vi "joystick+conversions.vi"(0 "Refnum in":refnum<k1>, 7 "error in (no error)":errorcluster, 8 "Stop":bool) -> (10 "dir info":i32, 12 "x axis info":i32, 13 "B pressed":bool, 14 "v_radial":dbl, 15 "y axis info":i32, 16 "A pressed":bool, 17 "y axis rot info":i32, 18 "chute":dbl, 19 "v_normal":dbl, 20 "Refnum out":refnum<k1>, 21 "X pressed":bool, 22 "R*w":dbl, 23 "Boolean":bool, 24 "z axis info (chute)":i32, 25 "Y pressed":bool, 26 "x axis rot info":i32, 27 "error out":errorcluster)   [LabVIEW 2016]
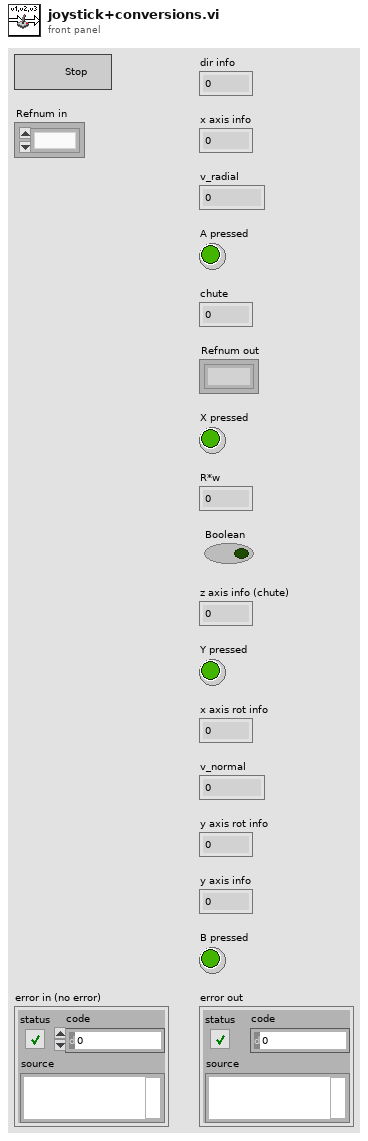
[diagram p1: front panel]
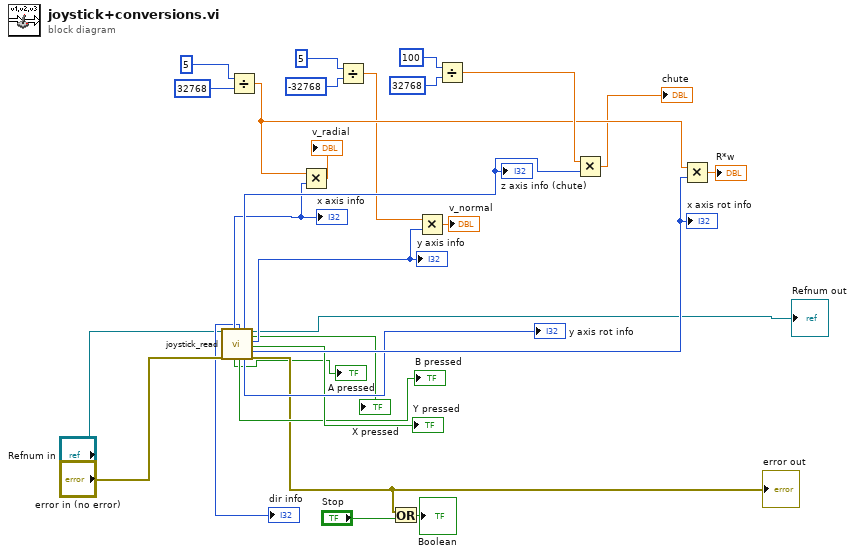
[diagram p0: block diagram]
diagram:
  n1 = call "joystick_read.vi"("Refnum in"="Refnum in", "error in (no error)"="error in (no error)") -> ("X axis"=w18:i32, "button 1"=→"A pressed":bool, "pov 1"=→"dir info":i32, "button 2"=→"B pressed":bool, "Z axis"=w26:i32, "Y axis rotation"=→"y axis rot info":i32, "Refnum out"=→"Refnum out":refnum<k1>, "button 3"=→"X pressed":bool, "Y axis"=w14:i32, "button 4"=→"Y pressed":bool, "X axis rotation"=w24:i32, "error out"=w8:errorcluster)  [unwired: 6 in]
  "x axis info" <- w18
  "y axis info" <- w14
  "z axis info (chute)" <- w26
  "x axis rot info" <- w24
  "error out" <- w8
  n2 = Divide(x=5, y=32768 ("x")) -> (x/y=w25:dbl)
  n3 = Multiply(x=w25, y=w18) -> (x*y=→"v_radial":dbl)
  n4 = Divide(x=5, y=-32768 ("x")) -> (x/y=w17:dbl)
  n5 = Or(x=w8, y="Stop") -> (x .or. y?=→"Boolean":bool)
  n6 = Multiply(x=w17, y=w14) -> (x*y=→"v_normal":dbl)
  n7 = Divide(x=100, y=32768 ("x")) -> (x/y=w28:dbl)
  n8 = Multiply(x=w28, y=w26) -> (x*y=→"chute":dbl)
  n9 = Multiply(x=w25, y=w24) -> (x*y=→"R*w":dbl)
